vi "_unstackArrayInner.vi"(8 "#iter":i32, 11 "Stacked Array":dbl[](array[numeric])) -> (3 "Unstacked Array":dbl[][](array[numeric]))   [LabVIEW 2021, in "System.lvclass"]
uses:
  System.lvclass
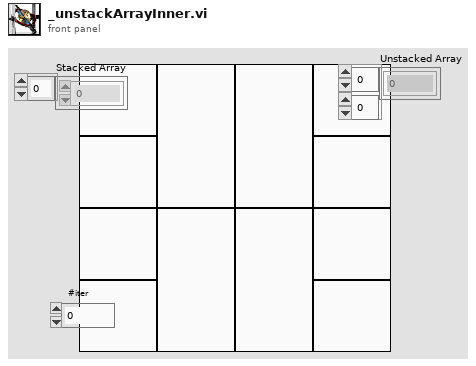
[diagram p1: front panel]
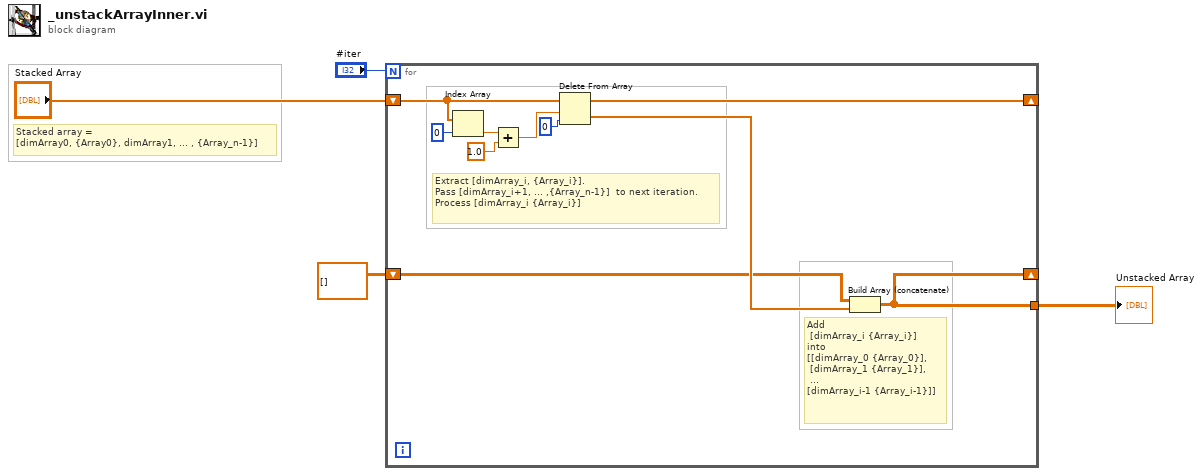
[diagram p0: block diagram]
diagram:
  # "Stacked array = \n[dimArray0, {Array0}, dimArray1, ... , {Array_n-1}]"
  n1 = for {
    N: "#iter" -> [_]
    shift-right: [w8] -> _
    shift-left: "Stacked Array" -> [w9]
    tunnel: [w5] -> w3
    shift-right: [w5] -> _
    shift-left: dbl[][] [] -> [w6]
    # "Add\n [dimArray_i {Array_i}]\ninto \n[[dimArray_0 {Array_0}],\n [dimArray_1 {Array_1}],\n ... \n[dimArray_i-1 {Array_i-1}]]"
    # "Extract [dimArray_i, {Array_i}].\nPass [dimArray_i+1, ... ,{Array_n-1}]  to next iteration.\nProcess [dimArray_i {Array_i}]"
    n2 = Index Array(array=w9, index=0) -> (element=w10:dbl)
    n3 = Add(x=w10, y=1.0) -> (x+y=w12:dbl)
    n4 = Delete From Array(array=w9, length=w12, index=0) -> (deleted portion=w7:dbl[], array with subset deleted=w8:dbl[])
    n5 = Build Array (concatenate)(w6, w7) -> (w5:dbl[][])
  }
  "Unstacked Array" <- w3
